vi "add element to configuration.vi"(4 "Module Runtime Objects":refnum<class "TBM module execution interface.lvclass">[](array[class]), 6 "Engine Runtime Object":refnum<class "Engine Runtime Interface.lvclass">, 8 "error in":errorcluster, 10 "engine configuration in":T1, 11 "Configuration in":T2[](array[typedef])) -> (0 "error out":errorcluster, 2 "engine loaded":string, 3 "Configuration out":T2[](array[typedef]))   [LabVIEW 2014, in "SMSLD TBD execution service.lvlib"]
uses:
  SMSLD TBD execution service.lvlib
  configuration elements.ctl
  <vilib>/NI/Module Execution Interface/Engine Configuration/engine configuration.lvclass
  <vilib>/NI/Module Execution Interface/Engine Runtime/Engine Runtime Interface.lvclass
  <vilib>/NI/Tag Bus Data Framework/Framework Configuration Classes/platypus configuration/engines cluster.ctl
  <vilib>/NI/Tag Bus Module Framework/module configuration/TBM module configuration.lvclass
  <vilib>/NI/Tag Bus Module Framework/runtime/TBM module execution interface.lvclass
  <vilib>/NI/Configuration Framework/serializable configuration/get alias.vi
  <vilib>/NI/Tag Bus Data Framework/Framework Configuration Classes/platypus configuration/PLConfigurationSerializer.lvlib
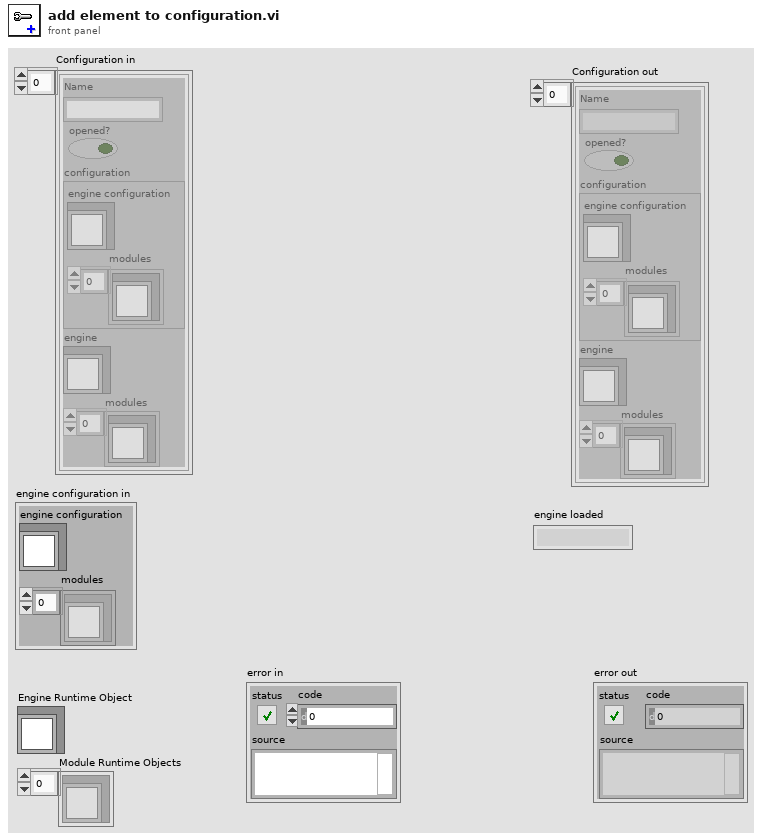
[diagram p1: front panel]
types:
  T1 = typedef "PLConfigurationSerializer.lvlib/engines cluster.ctl" = cluster{"engine configuration":refnum<class "engine configuration.lvclass">, "modules":refnum<class "TBM module configuration.lvclass">[]}
  T2 = typedef "SMSLD TBD execution service.lvlib/configuration elements.ctl" = cluster{"Name":string, "opened?":bool, "configuration":T1, "engine":refnum<class "Engine Runtime Interface.lvclass">, "modules":refnum<class "TBM module execution interface.lvclass">[]}
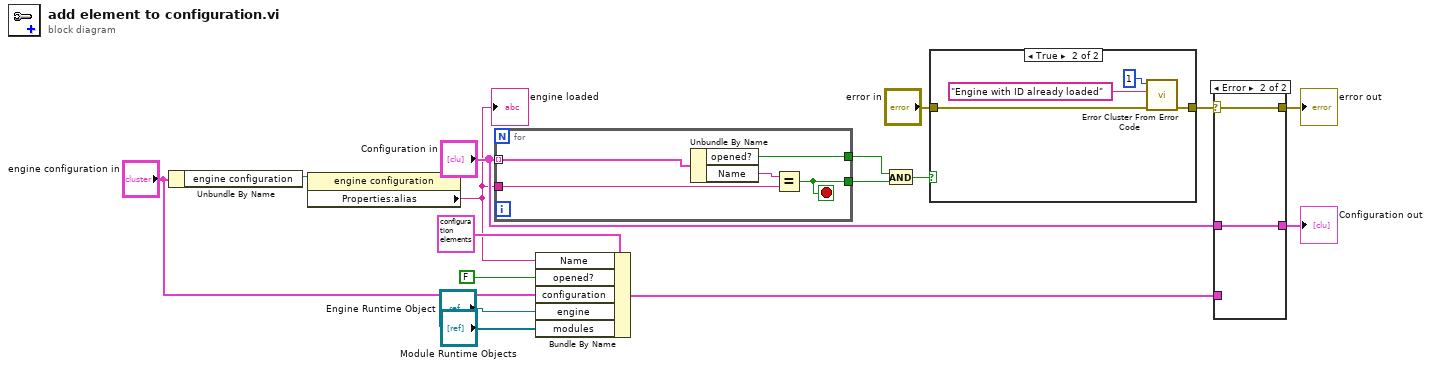
[diagram p0: block diagram]
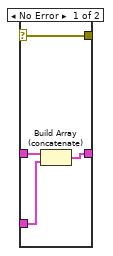
[diagram p2: hidden frame]
diagram:
  n1 = Unbundle By Name("engine configuration in") -> ("engine configuration"=w2:refnum<class "engine configuration.lvclass">)
  n2 = property class="engine configuration"(reference=w2) -> ("Properties:alias"=w1:string)  [unwired: 1 in, 2 out]
  "engine loaded" <- w1
  n3 = for {
    tunnel: "Configuration in" -> [w21] mode=indexing
    tunnel: w1 -> [w19]
    tunnel: [w18] -> w4
    tunnel: [w17] -> w6
    stop <- w17 stop-if-true
    n4 = Unbundle By Name(w21) -> ("opened?"=w18:bool, "Name"=w20:string)
    n5 = Equal?(x=w20, y=w19) -> (x = y?=w17:bool)
  }
  n6 = Bundle By Name(cluster=T2 {"Name"="", "opened?"=FALSE, "configuration"={"engine configuration"=refnum, "modules"=[]}, "engine"=refnum, "modules"=[]} ("configuration"), "Name"=w1, "opened?"=FALSE ("initialized?"), "configuration"="engine configuration in", "engine"="Engine Runtime Object", "modules"="Module Runtime Objects") -> (w7:T2)
  n7 = And(x=w4, y=w6) -> (x .and. y?=w5:bool)
  n8 = case shown="True" w5 {
    tunnel: [w22 w25] -> w15
    tunnel: "error in" -> [w22 w26]
    frame False {
    }
    frame True {
      n9 = call <vilib>:"Error Cluster From Error Code.vi"("error in (no error)"=w26, "error message (\"\")"="Engine with ID already loaded" ("error message (\"\")"), "error code (0)"=1) -> ("error out"=w25:errorcluster)  [unwired: 6 in]
    }
  }
  n10 = case shown="Error" w15 {
    selector: w15 -> [w28 w32]
    tunnel: [w28 w32] -> w14
    tunnel: "Configuration in" -> [w30 w31]
    tunnel: [w29 w31] -> w8
    tunnel: w7 -> [w27 _]
    frame No Error {
      n11 = Build Array (concatenate)(w30, w27) -> (w29:T2[])
    }
    frame Error {
    }
  }
  "Configuration out" <- w8
  "error out" <- w14
